vi "Reset_CAN.vi"(8 "error in (no error)":errorcluster, 9 "CAN 通道":u32(ring) items=["0", "1"], 10 "索引":u32(ring) items=["0", "1", "2", "3", "4", "5", "6", "7", "8"], 11 "设备类型":u32(ring)=3 items=["PCI5121"=1, "PCI9810"=2, "USBCAN1"=3, "USBCAN2"=4, "PCI9820"=5, "PCI5110"=7, "PC104CAN"=11, "CANETUDP"=12, "PCI9840B"=14, "PC104C2"=15, "PCI9820I"=16, "CANETTCP"=17, "PCIE9221"=24, "PCI5010U"=19, "USBCAN_E_U"=20, "USBCAN_2E_U"=21, "PCI5020U"=22, "PCIE9120I"=27, "PCIE9110I"=28, "PCIE9140I"=29]) -> (0 "error out":errorcluster)   [LabVIEW 2020, in "ZLG_CAN.lvlib"]
doc: "_____\nCreated using Delacor QMH Event Scripter 4.1.0.80."
uses:
  ZLG_CAN.lvlib
  Reset_CAN Argument--cluster.ctl
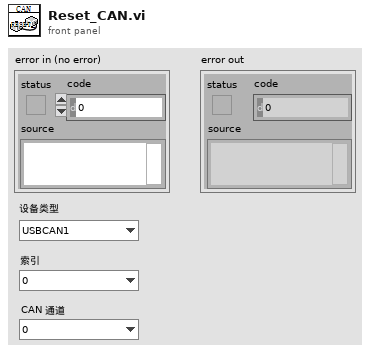
[diagram p1: front panel]
types:
  T1 = typedef "ZLG_CAN.lvlib/Reset_CAN Argument--cluster.ctl" = cluster{"设备类型":u32, "索引":u32, "CAN 通道":u32}
  T2 = typedef "ZLG_CAN.lvlib/Request Events--cluster.ctl" = cluster{"Stop Module":refnum<user-event>, "Show Panel":refnum<user-event>, "Hide Panel":refnum<user-event>, "Get Module Execution Status":refnum<user-event>, "Show Diagram":refnum<user-event>, "Open_CAN":refnum<user-event>, "Init_CAN":refnum<user-event>, "Start_CAN":refnum<user-event>, "Sent_CAN":refnum<user-event>, "Close_CAN":refnum<user-event>, "Reset_CAN":refnum<user-event>, "Recive_CAN":refnum<user-event>, "Recive_Wait":refnum<user-event>, "Sent_Recive":refnum<user-event>}
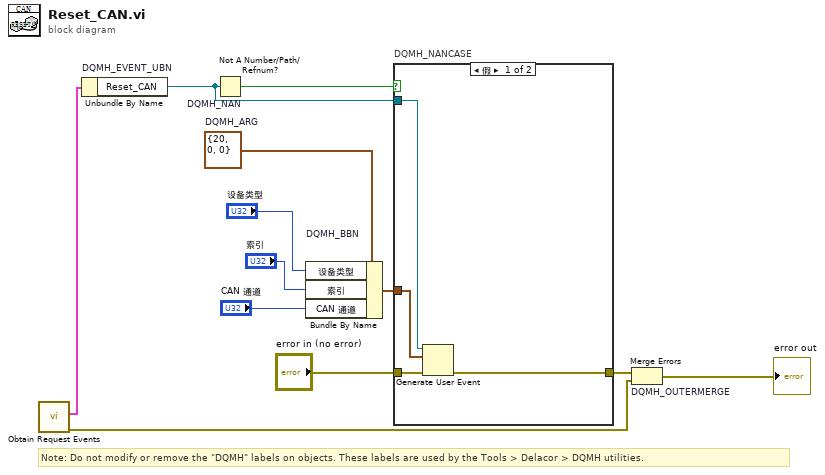
[diagram p0: block diagram]
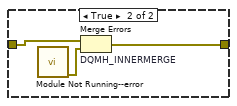
[diagram p2: hidden frame]
diagram:
  w6 = T1 {"设备类型"=20, "索引"=0, "CAN 通道"=0}  # DQMH_ARG
  # "Note: Do not modify or remove the \"DQMH\" labels on objects. These labels are used by the Tools > Delacor > DQMH utilities."
  n1 = call "Obtain Request Events.vi"() -> ("error out"=w5:errorcluster, "ZLG_CAN Request Events"=w4:T2)  [unwired: 10 in]
  n2 = Unbundle By Name "DQMH_EVENT_UBN"(w4) -> ("Reset_CAN"=w8:refnum<user-event>)
  n3 = Not A Number/Path/Refnum? "DQMH_NAN"(number/path/refnum=w8) -> (NaN/Path/Refnum?=w9:bool)
  n4 = Bundle By Name "DQMH_BBN"(cluster=w6, "设备类型"="设备类型", "索引"="索引", "CAN 通道"="CAN 通道") -> (w10:T1)
  n5 = case "DQMH_NANCASE" shown="假" w9 {
    tunnel: "error in (no error)" -> [w16 w19]
    tunnel: [w15 w18] -> w7
    tunnel: w8 -> [w14 _]
    tunnel: w10 -> [w13 _]
    frame False {
      n6 = Generate User Event(user event=w14, event data cluster=w13, error in=w16) -> (error out=w15:errorcluster)  [unwired: 1 in, 1 out]
    }
    frame True {
      n7 = call "Module Not Running--error.vi"() -> ("error out"=w17:errorcluster)  [unwired: 11 in]
      n8 = Merge Errors "DQMH_INNERMERGE"(w19, w17) -> (w18:errorcluster)
    }
  }
  n9 = Merge Errors "DQMH_OUTERMERGE"(w7, w5) -> (→"error out":errorcluster)
